vi "Add VI to Virtual Folder.vi"(7 "Virtual Folder":refnum<vi>, 8 "error in":errorcluster, 10 "VI Name":string, 11 "Path to VI":path) -> (0 "error out":errorcluster, 2 "VI Name":string, 3 "Path to VI":path)   [LabVIEW 2014, in "Initialization and IO Node Scripting.lvlib"]
uses:
  Initialization and IO Node Scripting.lvlib
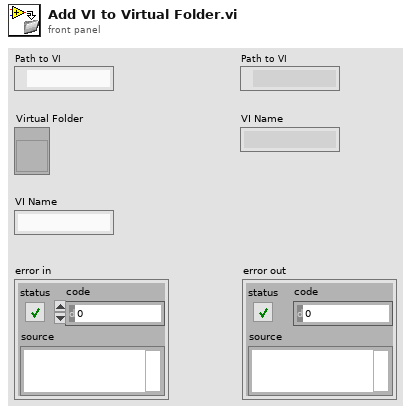
[diagram p1: front panel]
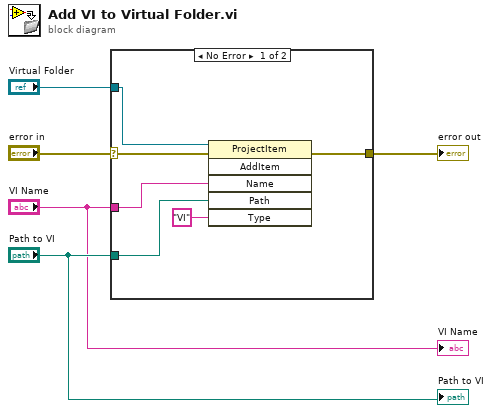
[diagram p0: block diagram]
diagram:
  n1 = case shown="No Error" "error in" {
    selector: "error in" -> [w9 w12]
    tunnel: "VI Name" -> [w10 _]
    tunnel: "Virtual Folder" -> [w8 _]
    tunnel: [w7 w12] -> w3
    tunnel: "Path to VI" -> [w6 _]
    frame No Error {
      n2 = invoke class="ProjectItem" method="AddItem"(reference=w8, error in=w9, "Name"=w10, "Path"=w6, "Type"="VI") -> (error out=w7:errorcluster)  [unwired: 1 in, 5 out]
    }
    frame Error {
    }
  }
  "error out" <- w3
  "Path to VI" <- "Path to VI"
  "VI Name" <- "VI Name"
